vi "Configure Save Waveform.vi"(0 "VISA resource name":refnum<visa-resource-name>, 1 "Trace Title (Title)":string="Title", 2 "Format (0: Binary)":u16(ring) items=["Binary", "ASCII", "Excel", "MATLAB", "MathCad", "WaveML"], 3 "SubFormat (1: Time & Amplitude)":u16(ring)=1 items=["Amplitude Only", "Time & Amplitude", "With Header"], 4 "BinarySubFormat (1: Word)":u16(ring)=1 items=["Byte", "Word", "Auto"], 5 "error in (no error)":errorcluster, 6 "Mode (0: Set All Properties)":T1(ring), 7 "Delimiter (  0:Comma)":u16(ring) items=["Comma", "Space", "Semicolon", "Tab"], 8 "Source (0: Channel 1)":u16(ring) items=["Channel 1", "Channel 2", "Channel 3", "Channel 4", "Memory 1", "Memory 2", "Memory 3", "Memory 4", "Function 1", "Function 2", "Function 3", "Function 4", "Function 5", "Function 6", "Function 7", "Function 8", "Other"], 9 "Save Files in Directory (D:\\Waveforms)":string="D:\\Waveforms", 10 "Custom Source ID":string, 11 "Auto Save (0:Off":u16(ring) items=["Off", "Wrap", "Fill"], 12 "Destination (0:File)":u16(ring) items=["File", "M1", "M2", "M3", "M4"]) -> (14 "VISA resource name out":refnum<visa-resource-name>, 19 "error out":errorcluster)   [LabVIEW 2015, in "LeCroy Wave Series.lvlib"]
doc: "This VI configures the controls in the Save Waveform setup screen. To store the waveform, use the VI 'Save Waveform.vi'"
uses:
  <instrlib>/LeCroy Wave Series/LeCroy Wave Series.lvlib
panel:
  # "Controls for Destination = File"
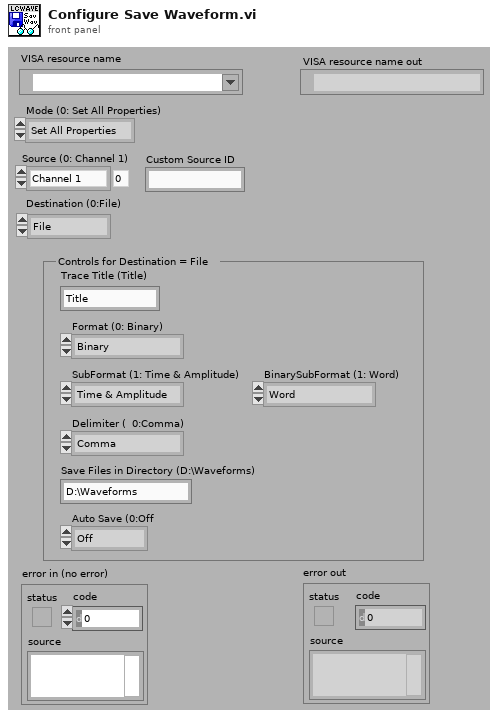
[diagram p1: front panel]
types:
  T1 = enum16{"Set All Properties", "Source", "Destination", "Trace Title", "Format", "SubFormat", "BinarySubFormat", "Delimiter", "FilePath", "AutoSave"}
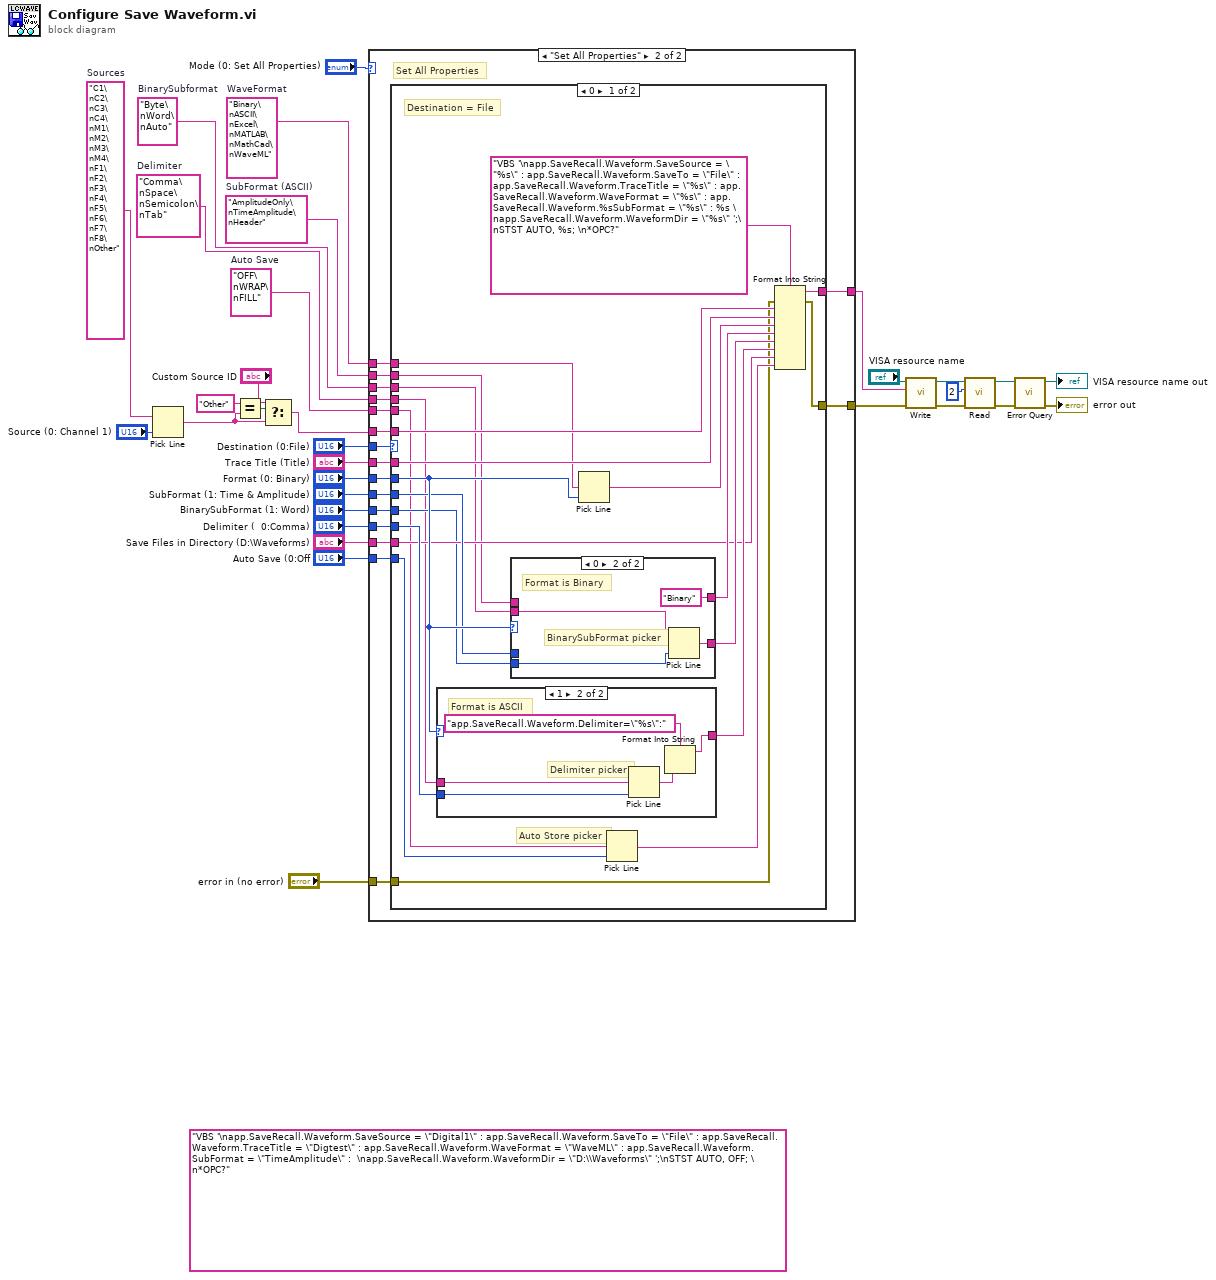
[diagram p0: block diagram]
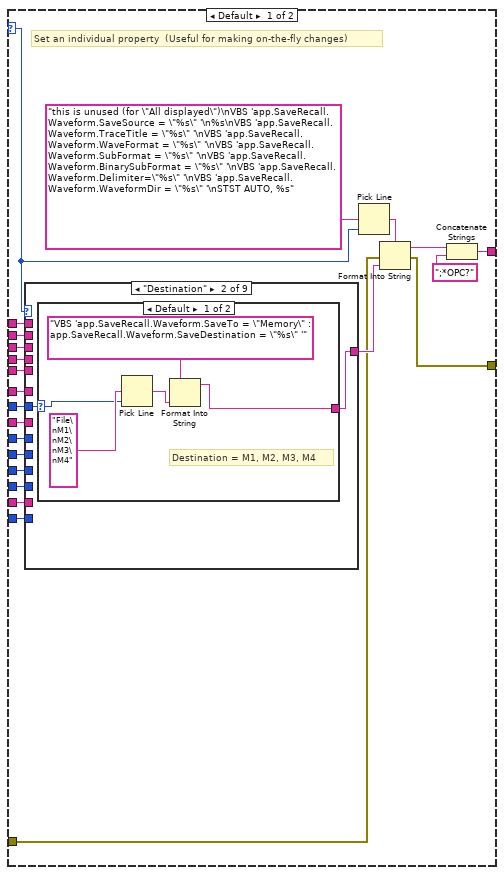
[diagram p2: hidden frame]
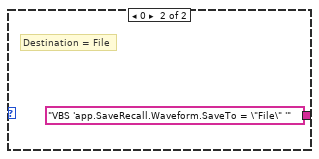
[diagram p4: hidden frame]
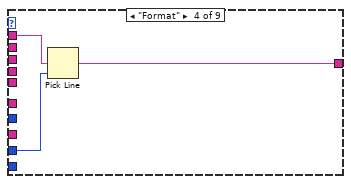
[diagram p6: hidden frame]
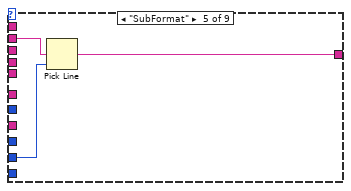
[diagram p7: hidden frame]
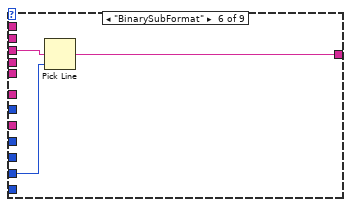
[diagram p8: hidden frame]
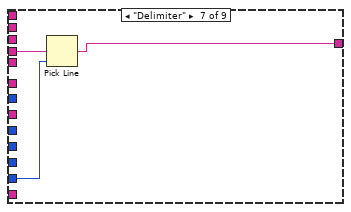
[diagram p9: hidden frame]
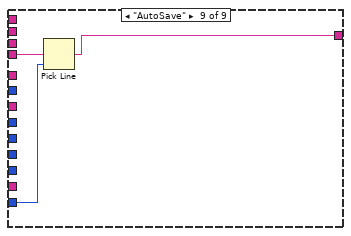
[diagram p11: hidden frame]
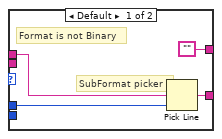
[diagram p13: hidden frame]
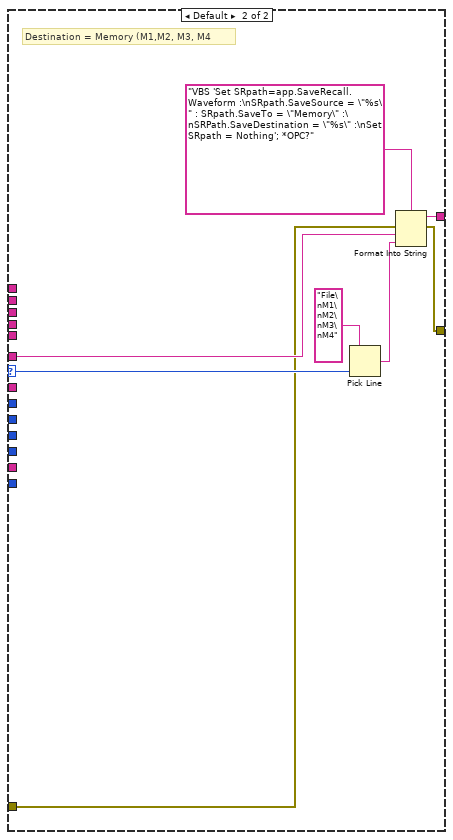
[diagram p14: hidden frame]
diagram:
  w5 = "C1\nC2\nC3\nC4\nM1\nM2\nM3\nM4\nF1\nF2\nF3\nF4\nF5\nF6\nF7\nF8\nOther"  # Sources
  (unwired) "VBS '\napp.SaveRecall.Waveform.SaveSource = \"Digital1\" : app.SaveRecall.Waveform.SaveTo = \"File\" : app.SaveRecall.Waveform.TraceTitle = \"Digtest\" : app.SaveRecall.Waveform.WaveFormat = \"WaveML\" : app.SaveRecall.Waveform.SubFormat = \"TimeAmplitude\" :  \napp.SaveRecall.Waveform.WaveformDir = \"D:\\Waveforms\" ';\nSTST AUTO, OFF; \n*OPC?" ("Write Buffer")
  w10 = "OFF\nWRAP\nFILL"  # Auto Save
  w11 = "Comma\nSpace\nSemicolon\nTab"  # Delimiter
  w12 = "Byte\nWord\nAuto"  # BinarySubformat
  w13 = "AmplitudeOnly\nTimeAmplitude\nHeader"  # SubFormat (ASCII)
  w14 = "Binary\nASCII\nExcel\nMATLAB\nMathCad\nWaveML"  # WaveFormat
  n1 = Pick Line(multi-line string=w5, line index="Source (0: Channel 1)") -> (output string=w2:string)  [unwired: 1 in]
  n2 = Equal?(x="Other", y=w2) -> (x = y?=w7:bool)
  n3 = Select(t="Custom Source ID", s=w7, f=w2) -> (s? t:f=w1:string)
  n4 = case shown="\"Set All Properties\"" "Mode (0: Set All Properties)" {
    selector: "Mode (0: Set All Properties)" -> [w45 _]
    tunnel: [w35 w98] -> w8
    tunnel: "Destination (0:File)" -> [w52 w97]
    tunnel: w1 -> [w53 w96]
    tunnel: "error in (no error)" -> [w42 w88]
    tunnel: [w41 w95] -> w25
    tunnel: "Trace Title (Title)" -> [w51 w94]
    tunnel: "Format (0: Binary)" -> [w50 w93]
    tunnel: "SubFormat (1: Time & Amplitude)" -> [w49 w92]
    tunnel: "Delimiter (  0:Comma)" -> [w48 w91]
    tunnel: "Save Files in Directory (D:\\Waveforms)" -> [w47 w90]
    tunnel: "Auto Save (0:Off" -> [w46 w89]
    tunnel: "BinarySubFormat (1: Word)" -> [w44 w87]
    tunnel: w14 -> [w40 w86]
    tunnel: w13 -> [w39 w85]
    tunnel: w12 -> [w38 w84]
    tunnel: w11 -> [w37 w83]
    tunnel: w10 -> [w36 w82]
    frame Default {
      # "Set an individual property  (Useful for making on-the-fly changes)"
      n5 = case shown="\"Destination\"" w45 {
        tunnel: w53 -> [w56 _ _ _ _ _ _ _ _]
        tunnel: w52 -> [_ w58 _ _ _ _ _ _ _]
        tunnel: w51 -> [_ _ w65 _ _ _ _ _ _]
        tunnel: w50 -> [_ _ _ w68 _ _ _ _ _]
        tunnel: w49 -> [_ _ _ _ w71 _ _ _ _]
        tunnel: w48 -> [_ _ _ _ _ _ w77 _ _]
        tunnel: w47 -> [_ _ _ _ _ _ _ w78 _]
        tunnel: w46 -> [_ _ _ _ _ _ _ _ w81]
        tunnel: w44 -> [_ _ _ _ _ w74 _ _ _]
        tunnel: [w56 w57 w65 w67 w70 w73 w76 w78 w80] -> w43
        tunnel: w40 -> [_ _ _ w66 _ _ _ _ _]
        tunnel: w39 -> [_ _ _ _ w69 _ _ _ _]
        tunnel: w38 -> [_ _ _ _ _ w72 _ _ _]
        tunnel: w37 -> [_ _ _ _ _ _ w75 _ _]
        tunnel: w36 -> [_ _ _ _ _ _ _ _ w79]
        frame "Source", Default {
        }
        frame "Destination" {
          n6 = case shown="Default" w58 {
            selector: w58 -> [w62 _]
            tunnel: [w59 "VBS 'app.SaveRecall.Waveform.SaveTo = \"File\" '"] -> w57
            frame Default {
              # "Destination = M1, M2, M3, M4"
              n7 = Pick Line(multi-line string="File\nM1\nM2\nM3\nM4", line index=w62) -> (output string=w61:string)  [unwired: 1 in]
              n8 = Format Into String(format string="VBS 'app.SaveRecall.Waveform.SaveTo = \"Memory\" : app.SaveRecall.Waveform.SaveDestination = \"%s\" '", w61) -> (resulting string=w59:string)  [unwired: 2 in, 1 out]
            }
            frame 0 {
              # "Destination = File"
            }
          }
        }
        frame "Trace Title" {
        }
        frame "Format" {
          n9 = Pick Line(multi-line string=w66, line index=w68) -> (output string=w67:string)  [unwired: 1 in]
        }
        frame "SubFormat" {
          n10 = Pick Line(multi-line string=w69, line index=w71) -> (output string=w70:string)  [unwired: 1 in]
        }
        frame "BinarySubFormat" {
          n11 = Pick Line(multi-line string=w72, line index=w74) -> (output string=w73:string)  [unwired: 1 in]
        }
        frame "Delimiter" {
          n12 = Pick Line(multi-line string=w75, line index=w77) -> (output string=w76:string)  [unwired: 1 in]
        }
        frame "FilePath" {
        }
        frame "AutoSave" {
          n13 = Pick Line(multi-line string=w79, line index=w81) -> (output string=w80:string)  [unwired: 1 in]
        }
      }
      n14 = Pick Line(multi-line string="this is unused (for \"All displayed\")\nVBS 'app.SaveRecall.Waveform.SaveSource = \"%s\" '\n%s\nVBS 'app.SaveRecall.Waveform.TraceTitle = \"%s\" '\nVBS 'app.SaveRecall.Waveform.WaveFormat = \"%s\" '\nVBS 'app.SaveRecall.Waveform.SubFormat = \"%s\" '\nVBS 'app.SaveRecall.Waveform.BinarySubFormat = \"%s\" '\nVBS 'app.SaveRecall.Waveform.Delimiter=\"%s\" '\nVBS 'app.SaveRecall.Waveform.WaveformDir = \"%s\" '\nSTST AUTO, %s", line index=w45) -> (output string=w54:string)  [unwired: 1 in]
      n15 = Format Into String(format string=w54, error in=w42, w43) -> (resulting string=w34:string, error out=w41:errorcluster)  [unwired: 1 in]
      n16 = Concatenate Strings(w34, ";*OPC?") -> (w35:string)
    }
    frame "Set All Properties" {
      # "Set All Properties"
      n17 = case shown="0" w97 {
        selector: w97 -> [_ w138]
        tunnel: [w120 w141] -> w98
        tunnel: w96 -> [w119 w136]
        tunnel: [w117 w135] -> w95
        tunnel: w94 -> [w111 _]
        tunnel: w93 -> [w110 _]
        tunnel: w92 -> [w109 _]
        tunnel: w91 -> [w108 _]
        tunnel: w90 -> [w107 _]
        tunnel: w89 -> [w106 _]
        tunnel: w88 -> [w105 w134]
        tunnel: w87 -> [w104 _]
        tunnel: w86 -> [w103 _]
        tunnel: w85 -> [w102 _]
        tunnel: w84 -> [w101 _]
        tunnel: w83 -> [w100 _]
        tunnel: w82 -> [w99 _]
        frame 0 {
          # "Destination = File"
          # "Auto Store picker"
          n18 = case shown="1" w110 {
            tunnel: [_ w123] -> w112
            tunnel: w108 -> [_ w122]
            tunnel: w100 -> [_ w121]
            frame Default {
            }
            frame 1 {
              # "Delimiter picker"
              # "Format is ASCII"
              n19 = Pick Line(multi-line string=w121, line index=w122) -> (output string=w124:string)  [unwired: 1 in]
              n20 = Format Into String(format string="app.SaveRecall.Waveform.Delimiter=\"%s\":", w124) -> (resulting string=w123:string)  [unwired: 2 in, 1 out]
            }
          }
          n21 = case shown="0" w110 {
            tunnel: ["" "Binary"] -> w115
            tunnel: [w128 w132] -> w114
            tunnel: w109 -> [w127 _]
            tunnel: w104 -> [_ w131]
            tunnel: w102 -> [w126 _]
            tunnel: w101 -> [_ w130]
            frame Default {
              # "SubFormat picker"
              # "Format is not Binary"
              n22 = Pick Line(multi-line string=w126, line index=w127) -> (output string=w128:string)  [unwired: 1 in]
            }
            frame 0 {
              # "BinarySubFormat picker"
              # "Format is Binary"
              n23 = Pick Line(multi-line string=w130, line index=w131) -> (output string=w132:string)  [unwired: 1 in]
            }
          }
          n24 = Pick Line(multi-line string=w103, line index=w110) -> (output string=w116:string)  [unwired: 1 in]
          n25 = Pick Line(multi-line string=w99, line index=w106) -> (output string=w113:string)  [unwired: 1 in]
          n26 = Format Into String(format string="VBS '\napp.SaveRecall.Waveform.SaveSource = \"%s\" : app.SaveRecall.Waveform.SaveTo = \"File\" : app.SaveRecall.Waveform.TraceTitle = \"%s\" : app.SaveRecall.Waveform.WaveFormat = \"%s\" : app.SaveRecall.Waveform.%sSubFormat = \"%s\" : %s \napp.SaveRecall.Waveform.WaveformDir = \"%s\" ';\nSTST AUTO, %s; \n*OPC?", error in=w105, w119, w111, w116, w115, w114, w112, w107, w113) -> (resulting string=w120:string, error out=w117:errorcluster)  [unwired: 1 in]
        }
        frame Default {
          # "Destination = Memory (M1,M2, M3, M4"
          n27 = Pick Line(multi-line string="File\nM1\nM2\nM3\nM4", line index=w138) -> (output string=w137:string)  [unwired: 1 in]
          n28 = Format Into String(format string="VBS 'Set SRpath=app.SaveRecall.Waveform :\nSRpath.SaveSource = \"%s\" : SRpath.SaveTo = \"Memory\" :\nSRPath.SaveDestination = \"%s\" :\nSet SRpath = Nothing'; *OPC?", error in=w134, w136, w137) -> (resulting string=w141:string, error out=w135:errorcluster)  [unwired: 1 in]
        }
      }
    }
  }
  n29 = call <instrlib>:"Write.vi"("error in (no error)"=w25, "Write Buffer"=w8, "VISA resource name"="VISA resource name") -> ("error out"=w29:errorcluster, "VISA resource name out"=w30:refnum<visa-resource-name>)  [unwired: 6 in, 1 out]
  n30 = call <instrlib>:"Read.vi"("error in (no error)"=w29, "Byte Count"=u32 2, "VISA resource name"=w30) -> ("error out"=w28:errorcluster, "VISA resource name out"=w23:refnum<visa-resource-name>)  [unwired: 5 in, 2 out]
  n31 = call <instrlib>:"Error Query.vi"("error in (no error)"=w28, "VISA resource name"=w23) -> ("error out"=→"error out":errorcluster, "VISA resource name out"=→"VISA resource name out":refnum<visa-resource-name>)  [unwired: 6 in, 2 out]
